vi "hdt_build_stream_sicm.vi"(11 "readyForOutput":bool[](array[boolean])=[FALSE, FALSE, FALSE, FALSE, FALSE, FALSE, FALSE]) -> (3 "dataStream":cluster{fxp<+/-,22,1>[], bool[]})   [LabVIEW 2016]
uses:
  <vilib>/rvi/Emulation/niFpgaEmulationIsFPGAContextNoSignature.vi
  <vilib>/rvi/Emulation/niFpgaSctlEmulationGetInTimedLoop.vi
  <vilib>/rvi/errors/niFpgaSetErrorForExecOnDevCompSimple.vi
  <vilib>/rvi/eio/common/nirviEmuReportErrorAndStop.vi
  <vilib>/rvi/DataTransferAndStorage/Container/Common/niFpgaContainerGetUniqueNameForEmu.vi
  <vilib>/rvi/FIFO/Fifo_Resource/nirvififoEmulationSetSize.vi
  <vilib>/rvi/FIFO/Fifo_Resource/nirviFifoEmulationQueueMgr.vi
  <instcachedir>/0/nirviFifoEmulationQueueMgr_E5CAEC123FF24DC58D834DCA3CDAA9B5.lvgen/nirviFifoEmulationQueueMgr_E5CAEC123FF24DC58D834DCA3CDAA9B5_032.vi
  <vilib>/Utility/error.llb/Clear Errors.vi
  <vilib>/rvi/FIFO/Fifo_Resource/nirvififoEmulationCreateLock.vi
  <vilib>/rvi/Emulation/niFpgaProcessEmulError.vi
  <vilib>/rvi/FIFO/Fifo_Resource/nirvififoEmulationObtainLock.vi
  <vilib>/rvi/FIFO/Fifo_Resource/nirvififoEmulationReleaseLock.vi
  <vilib>/rvi/occurrence/nirviWaitOnOccurrenceBase.vi
  <vilib>/rvi/errors/nirviReportUnexpectedCaseInternalError.vi
  <vilib>/rvi/errors/nirviReportUnexpectedCaseInternalError (U32).vi
  <instcachedir>/0/nirviFifoEmulationQueueMgr_E5CAEC123FF24DC58D834DCA3CDAA9B5.lvgen/nirviFifoEmulationQueueMgr_E5CAEC123FF24DC58D834DCA3CDAA9B5_000.vi
  <vilib>/rvi/DataTransferAndStorage/Container/XNode/niFpgaContainer.xnode
  <vilib>/rvi/FIFO/Fifo_Resource/nirvififoEmulationRead.vi
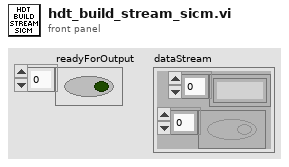
[diagram p1: front panel]
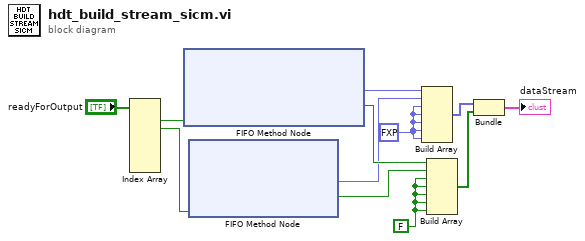
[diagram p0: block diagram]
diagram:
  w5 = fxp<+/-,24,16> 0.0 ("element")
  w6 = FALSE
  n1 = Index Array(array="readyForOutput") -> (element #1=w8:bool, element #2=w1:bool)  [unwired: 7 in, 5 out]
  n2 = xnode ("FIFO Method Node")("Ready for Output"=w8) -> ("Element"=w9:fxp<+/-,22,4>, "Output Valid"=w7:bool)  [unwired: 1 in, 1 out]
  n3 = xnode ("FIFO Method Node")("Ready for Output"=w1) -> ("Element"=w3:fxp<+/-,24,16>, "Output Valid"=w2:bool)  [unwired: 1 in, 1 out]
  n4 = Build Array(w9, w3, w5, w5, w5, w5, w5) -> (w10:fxp<+/-,34,16>[])
  n5 = Build Array(w7, w2, w6, w6, w6, w6, w6) -> (w11:bool[])
  n6 = Bundle(w10, w11) -> (→"dataStream":cluster{fxp<+/-,34,16>[], bool[]})  [unwired: 1 in]
